vi "Build State Machine.vi"() -> ()   [LabVIEW 2019, in "VIPM.lvclass"]
uses:
  VIPM.lvclass
  <vilib>/Utility/sysdir.llb/System Directory Type.ctl
  <vilib>/Utility/file.llb/Read Delimited Spreadsheet (string).vi
  <vilib>/Utility/file.llb/Write Delimited Spreadsheet (string).vi
  <vilib>/JKI/VIPM API/VIPM API_vipm_api.lvlib
panel:
  out "Selected List":string
  in  "Publish":bool
  in  "Choose File":bool
  in  "Open Selected":bool
  in  "Preview All":bool
  in  "Build All":bool
  in  "Build Selected":bool
  in  "Preview Selected":bool
  out "Status":string
  in  "File List":i32(listbox)
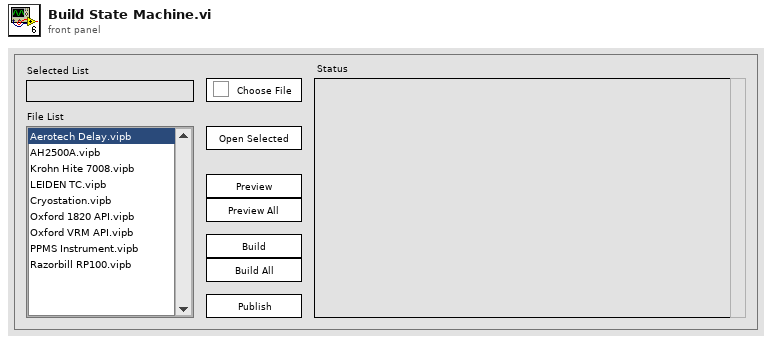
[diagram p1: front panel]
types:
  T1 = enum32{"Invalid", "Standard", "Closed", "Hidden", "Minimized", "Maximized"}
  T2 = enum32{"invalid app kind", "Development System", "Run Time System", "Student Edition", "Embedded LabVIEW", "Evaluation", "Custom"}
  T3 = enum8{"Enabled", "Disabled", "Disabled and Grayed Out"}
  T4 = cluster{"Core":cluster{"Current VI Reference":refnum<vi>, "Close Panel on Exit?":bool}, "lvproj paths":path[], "vipb paths":path[], "vip paths":path[], "selected path":path, "config path":path}
  T5 = typedef "System Directory Type.ctl" = i32
  T6 = cluster{"Current VI Reference":refnum<vi>, "Close Panel on Exit?":bool}
  T7 = typedef "VIPM API_vipm_api.lvlib/VI Package Build Spec Data Cluster_vipm_api.ctl" = cluster{"Package Version":T8, "Product Name":string, "Company Name":string, "Author Name (Person or Company)":string, "Product Homepage (URL)":string, "Legal Copyright":string, "License Agreement Name":string, "Product Description Summary":string, "Product Description":string, "Release Notes - Change Log":string}
  T8 = typedef "VIPM API_vipm_api.lvlib/Version Info Cluster_vipm_api.ctl" = cluster{"major":u32, "minor":u32, "patch":u32, "build":u32}
  T9 = typedef "VIPM API_vipm_api.lvlib/Repository Info Cluster_vipm_api.ctl" = cluster{"Repository Name":string, "Repository Folder Location":path}
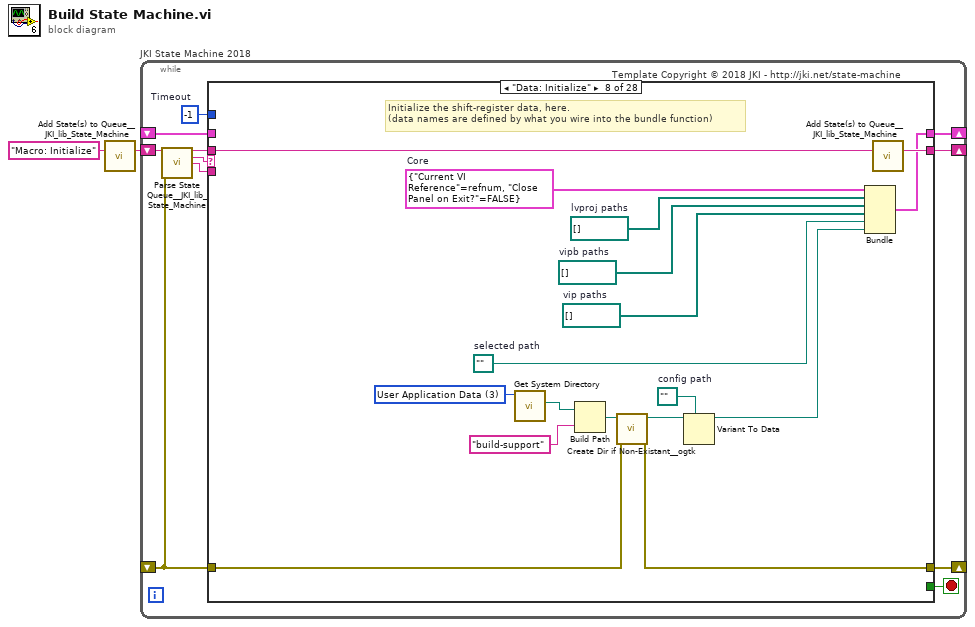
[diagram p0: block diagram]
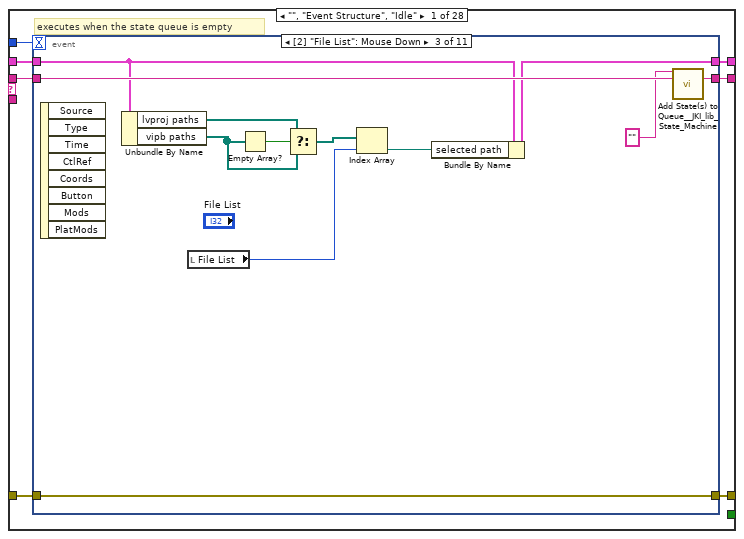
[diagram p2: hidden frame]
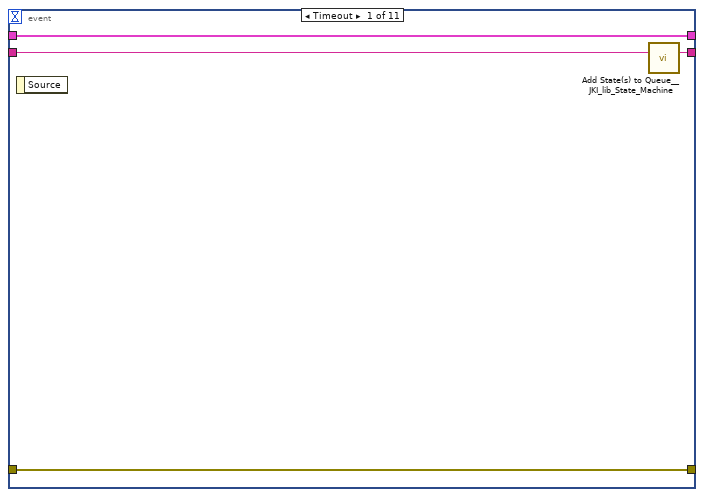
[diagram p3: hidden frame]
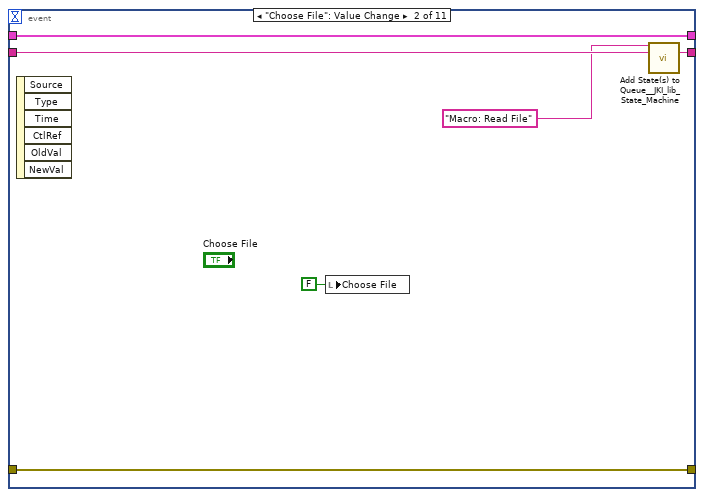
[diagram p4: hidden frame]
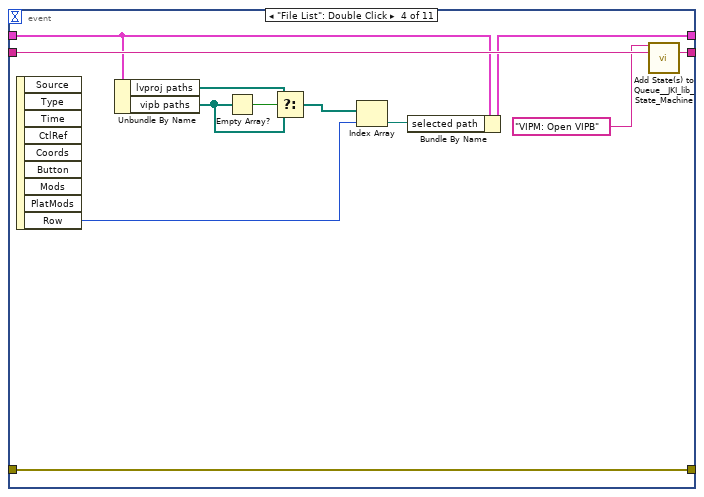
[diagram p5: hidden frame]
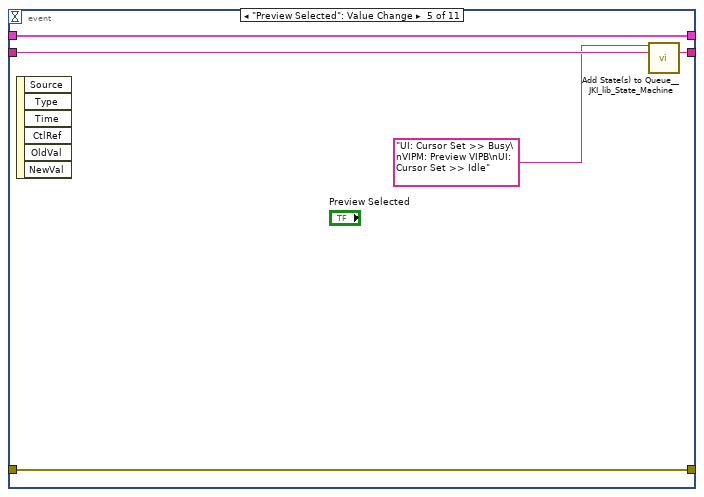
[diagram p6: hidden frame]
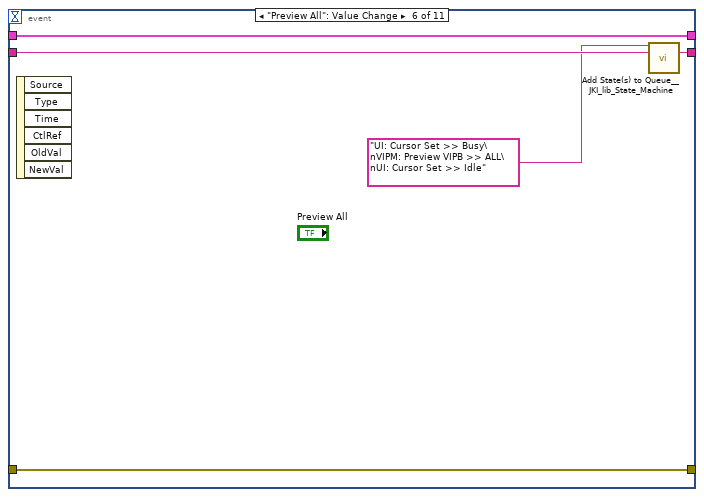
[diagram p7: hidden frame]
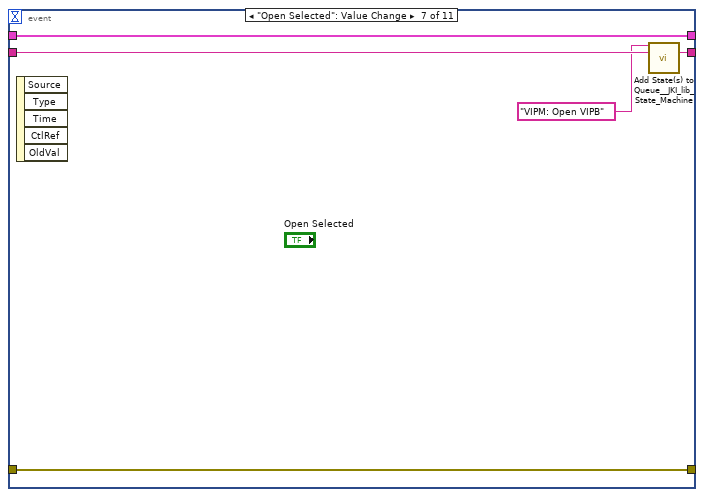
[diagram p8: hidden frame]
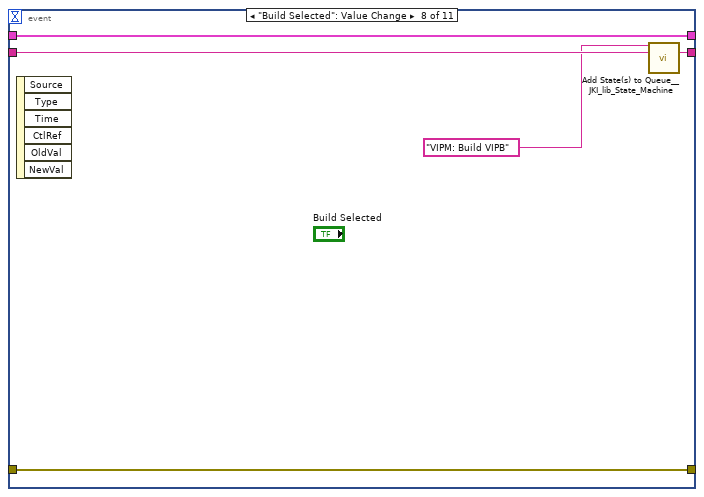
[diagram p9: hidden frame]
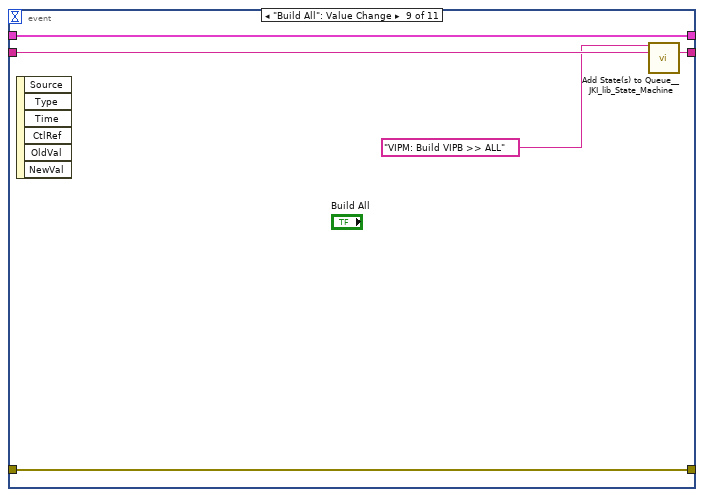
[diagram p10: hidden frame]
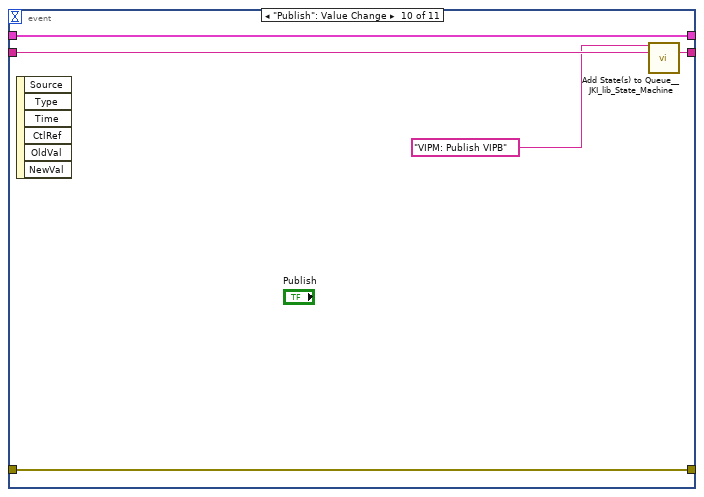
[diagram p11: hidden frame]
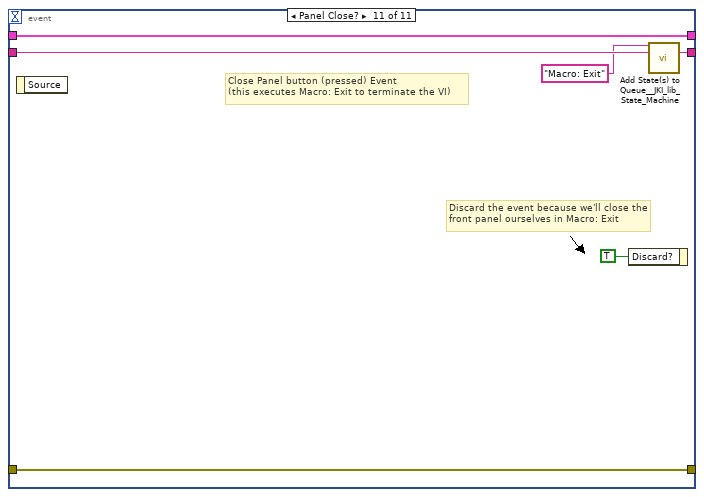
[diagram p12: hidden frame]
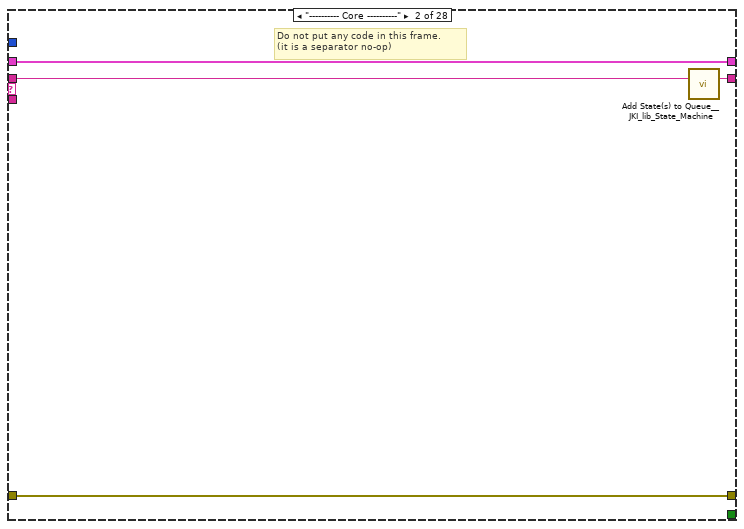
[diagram p13: hidden frame]
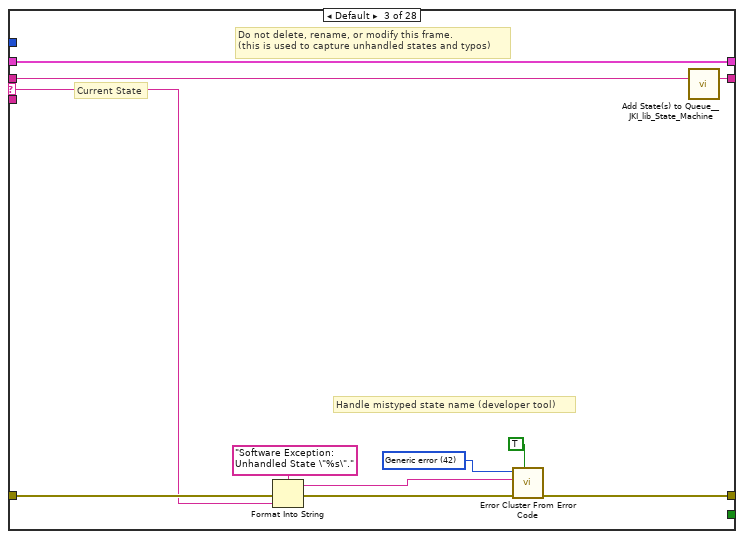
[diagram p14: hidden frame]
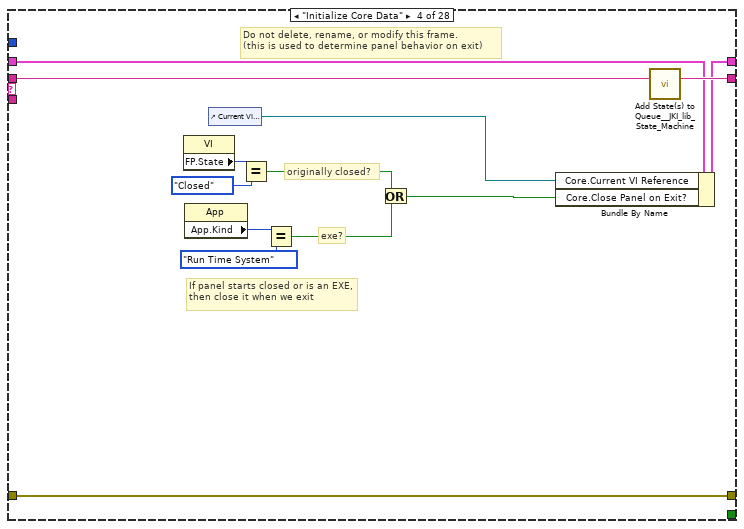
[diagram p15: hidden frame]
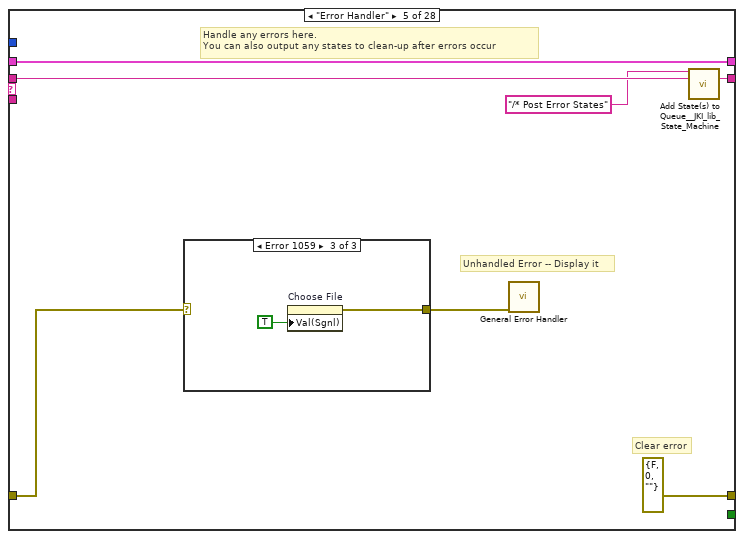
[diagram p16: hidden frame]
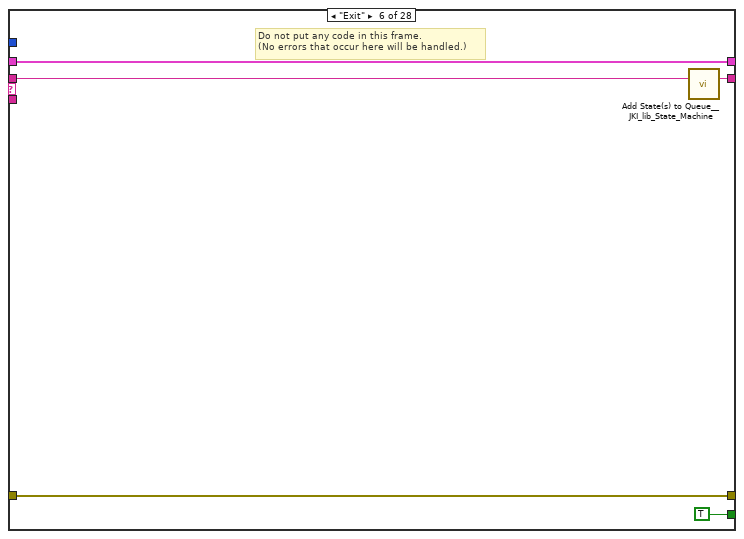
[diagram p19: hidden frame]
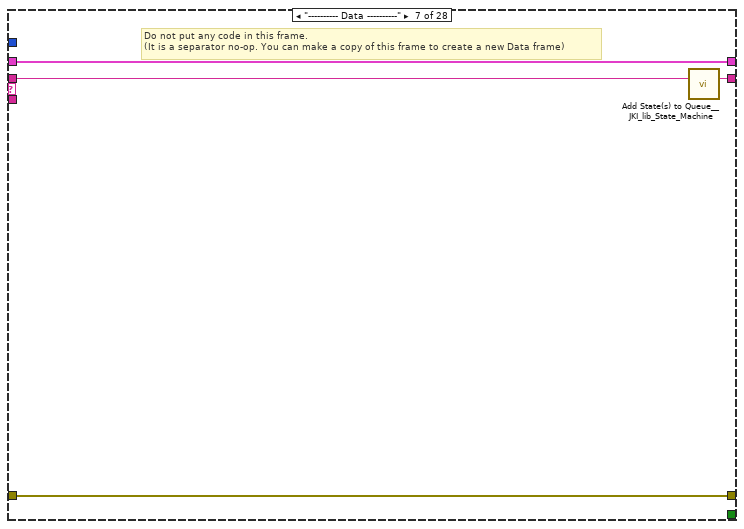
[diagram p20: hidden frame]
diagram:
  n1 = call <vilib>:"Add State(s) to Queue__JKI_lib_State_Machine.vi"("State(s) in (\"\")"="Macro: Initialize") -> ("States Out"=w2:string)  [unwired: 14 in]
  n2 = while "JKI State Machine 2018" {
    shift-right: [w6] -> _
    shift-left: _ -> [w5]
    shift-right: [w9] -> _
    shift-left: _ -> [w3]
    shift-right: [w8] -> _
    shift-left: w2 -> [w10]
    stop <- w7 stop-if-true
    w4 = -1  # Timeout
    # "Template Copyright © 2018 JKI - http://jki.net/state-machine"
    n3 = call <vilib>:"Parse State Queue__JKI_lib_State_Machine.vi"("State Queue"=w10, "Error In (no error)"=w3) -> ("Remaining States"=w12:string, "Current State"=w13:string, "Arguments"=w11:string)  [unwired: 11 in]
    n4 = case shown="\"Data: Initialize\"" w13 {
      selector: w13 -> [_ _ w95 _ _ _ _ _ _ _ _ _ _ _ _ _ _ _ _ _ _ _ _ _ _ _ _ _]
      tunnel: w12 -> [w20 w94 w99 w118 w125 w134 w138 w155 w161 w173 w186 w207 w226 w230 w236 w247 w264 w272 w283 w352 w357 w362 w372 w376 w389 w403 w426 w443]
      tunnel: w11 -> [_ _ _ _ _ _ _ _ _ _ _ _ _ _ _ _ _ w267 w277 _ _ _ _ _ _ w397 w412 _]
      tunnel: w5 -> [w18 w91 w97 w111 w122 w132 w135 _ w156 w165 w179 w204 w224 w227 w234 w244 w255 w270 w279 w349 w354 w359 w369 w373 w387 w400 w415 w437]
      tunnel: [w17 w92 w101 w115 errorcluster {"status"=FALSE, "code"=0, "source"=""} ("error out") w131 w136 w147 w157 w171 w176 w193 w220 w228 w233 w245 w262 w268 w280 w350 w355 w360 w370 w374 w382 w399 w418 w435] -> w9
      tunnel: w3 -> [w16 w92 w100 w115 w120 w131 w136 w146 w158 w171 w181 w202 w221 w228 w232 w245 w262 w269 w281 w350 w355 w360 w370 w374 w381 w398 w417 w434]
      tunnel: [w19 w93 w98 w117 w124 w133 w137 w154 w160 w172 w185 w206 w225 w229 w235 w246 w263 w271 w282 w351 w356 w361 w371 w375 w388 w402 w425 w442] -> w8
      tunnel: [_ _ _ _ _ TRUE _ _ _ _ _ _ _ _ _ _ _ _ _ _ _ _ _ _ _ _ _ _] -> w7
      tunnel: [w15 w91 w97 w116 w122 w132 w135 w153 w156 w166 w180 w205 w224 w227 w234 w244 w255 w270 w279 w349 w354 w359 w369 w373 w387 w400 w416 w437] -> w6
      tunnel: w4 -> [w14 _ _ _ _ _ _ _ _ _ _ _ _ _ _ _ _ _ _ _ _ _ _ _ _ _ _ _]
      frame "", "Event Structure", "Idle" {
        # "executes when the state queue is empty"
        n5 = event shown="[2] \"File List\": Mouse Down" {
          selector: _ -> [_ _ _ _ _ _ _ _ _ _ _]
          dyn-events: _ -> [_ _ _ _ _ _ _ _ _ _ _]
          timeout: w14 -> [_ _ _ _ _ _ _ _ _ _ _]
          tunnel: w20 -> [w24 w30 w42 w54 w59 w64 w69 w74 w79 w84 w90]
          tunnel: [w23 w29 w41 w53 w58 w63 w68 w73 w78 w83 w89] -> w19
          tunnel: w18 -> [w21 w25 w39 w44 w56 w61 w65 w71 w76 w81 w87]
          tunnel: [w22 w26 w40 w52 w57 w62 w67 w72 w77 w82 w88] -> w17
          tunnel: w16 -> [w22 w26 w40 w52 w57 w62 w67 w72 w77 w82 w88]
          tunnel: [w21 w25 w38 w51 w56 w61 w65 w71 w76 w81 w87] -> w15
          event Timeout {
            n6 = event-data() -> ()  [unwired: 1 in, 1 out]
            n7 = call <vilib>:"Add State(s) to Queue__JKI_lib_State_Machine.vi"("State(s) in (\"\")"=w24) -> ("States Out"=w23:string)  [unwired: 14 in]
          }
          event "Choose File": Value Change {
            n8 = event-data() -> ()  [unwired: 1 in, 6 out]
            n9 = local write "Choose File"(FALSE ("Choose File")) -> ()
            n10 = call <vilib>:"Add State(s) to Queue__JKI_lib_State_Machine.vi"("State(s) in Front (\"\")"="Macro: Read File" ("State(s) in Front (\"\")"), "State(s) in (\"\")"=w30) -> ("States Out"=w29:string)  [unwired: 13 in]
          }
          event "File List": Mouse Down {
            n11 = event-data() -> ()  [unwired: 1 in, 8 out]
            n12 = Unbundle By Name(w39) -> ("lvproj paths"=w33:path[], "vipb paths"=w31:path[])
            n13 = local read "File List"() -> (w35:i32)
            n14 = Empty Array?(array=w31) -> (empty?=w34:bool)
            n15 = Select(t=w33, s=w34, f=w31) -> (s? t:f=w32:path[])
            n16 = Index Array(array=w32, index=w35) -> (element=w37:path)
            n17 = Bundle By Name(cluster=w39, "selected path"=w37) -> (w38:T4)
            n18 = call <vilib>:"Add State(s) to Queue__JKI_lib_State_Machine.vi"("State(s) in Front (\"\")"="" ("State(s) in Front (\"\")"), "State(s) in (\"\")"=w42) -> ("States Out"=w41:string)  [unwired: 13 in]
          }
          event "File List": Double Click {
            n19 = event-data() -> ("Row"=w43:i32)  [unwired: 1 in, 8 out]
            n20 = Unbundle By Name(w44) -> ("lvproj paths"=w47:path[], "vipb paths"=w46:path[])
            n21 = Empty Array?(array=w46) -> (empty?=w48:bool)
            n22 = Select(t=w47, s=w48, f=w46) -> (s? t:f=w45:path[])
            n23 = Index Array(array=w45, index=w43) -> (element=w50:path)
            n24 = Bundle By Name(cluster=w44, "selected path"=w50) -> (w51:T4)
            n25 = call <vilib>:"Add State(s) to Queue__JKI_lib_State_Machine.vi"("State(s) in Front (\"\")"="VIPM: Open VIPB" ("State(s) in Front (\"\")"), "State(s) in (\"\")"=w54) -> ("States Out"=w53:string)  [unwired: 13 in]
          }
          event "Preview Selected": Value Change {
            n26 = event-data() -> ()  [unwired: 1 in, 6 out]
            n27 = call <vilib>:"Add State(s) to Queue__JKI_lib_State_Machine.vi"("State(s) in Front (\"\")"="UI: Cursor Set >> Busy\nVIPM: Preview VIPB\nUI: Cursor Set >> Idle" ("State(s) in Front (\"\")"), "State(s) in (\"\")"=w59) -> ("States Out"=w58:string)  [unwired: 13 in]
          }
          event "Preview All": Value Change {
            n28 = event-data() -> ()  [unwired: 1 in, 6 out]
            n29 = call <vilib>:"Add State(s) to Queue__JKI_lib_State_Machine.vi"("State(s) in Front (\"\")"="UI: Cursor Set >> Busy\nVIPM: Preview VIPB >> ALL\nUI: Cursor Set >> Idle" ("State(s) in Front (\"\")"), "State(s) in (\"\")"=w64) -> ("States Out"=w63:string)  [unwired: 13 in]
          }
          event "Open Selected": Value Change {
            n30 = event-data() -> ()  [unwired: 1 in, 5 out]
            n31 = call <vilib>:"Add State(s) to Queue__JKI_lib_State_Machine.vi"("State(s) in Front (\"\")"="VIPM: Open VIPB" ("State(s) in Front (\"\")"), "State(s) in (\"\")"=w69) -> ("States Out"=w68:string)  [unwired: 13 in]
          }
          event "Build Selected": Value Change {
            n32 = event-data() -> ()  [unwired: 1 in, 6 out]
            n33 = call <vilib>:"Add State(s) to Queue__JKI_lib_State_Machine.vi"("State(s) in Front (\"\")"="VIPM: Build VIPB" ("State(s) in Front (\"\")"), "State(s) in (\"\")"=w74) -> ("States Out"=w73:string)  [unwired: 13 in]
          }
          event "Build All": Value Change {
            n34 = event-data() -> ()  [unwired: 1 in, 6 out]
            n35 = call <vilib>:"Add State(s) to Queue__JKI_lib_State_Machine.vi"("State(s) in Front (\"\")"="VIPM: Build VIPB >> ALL" ("State(s) in Front (\"\")"), "State(s) in (\"\")"=w79) -> ("States Out"=w78:string)  [unwired: 13 in]
          }
          event "Publish": Value Change {
            n36 = event-data() -> ()  [unwired: 1 in, 6 out]
            n37 = call <vilib>:"Add State(s) to Queue__JKI_lib_State_Machine.vi"("State(s) in Front (\"\")"="VIPM: Publish VIPB" ("State(s) in Front (\"\")"), "State(s) in (\"\")"=w84) -> ("States Out"=w83:string)  [unwired: 13 in]
          }
          event Panel Close? {
            # "Discard the event because we'll close the front panel ourselves in Macro: Exit"
            # "Close Panel button (pressed) Event\n(this executes Macro: Exit to terminate the VI)"
            n38 = event-data() -> ()  [unwired: 1 in, 1 out]
            n39 = event-data("Discard?"=TRUE) -> ()  [unwired: 1 in, 1 out]
            n40 = call <vilib>:"Add State(s) to Queue__JKI_lib_State_Machine.vi"("State(s) in Front (\"\")"="Macro: Exit", "State(s) in (\"\")"=w90) -> ("States Out"=w89:string)  [unwired: 13 in]
          }
        }
      }
      frame "---------- Core ----------" {
        # "Do not put any code in this frame.\n(it is a separator no-op)"
        n41 = call <vilib>:"Add State(s) to Queue__JKI_lib_State_Machine.vi"("State(s) in (\"\")"=w94) -> ("States Out"=w93:string)  [unwired: 14 in]
      }
      frame Default {
        w104 = 42 items=["No error", "Argument error", "Memory is full", "Out of zone", "End of file", "File already open", "Generic file I/O error", "File not found", "File permission error", "Disk is full", "Duplicate path", "Too many files open", "System feature not enabled", "Resource file not found", "Cannot add resource", "Resource not found", "Image not found", "Image memory error", "Pen does not exist", "Config type invalid", "Config token not found", "Config parse error", "Config memory error", "Bad external code format", "Bad external code offset", "External code not present", "Null window", "Destroy window error", "Null menu", "Print aborted", "Bad print record", "Print driver error", "Windows error during printing", "Memory error during printing", "Print dialog error", "Generic print error", "Invalid device refnum", "Device not found", "Device parameter error", "Device unit error", "Cannot open device", "Device call aborted", "Generic error", "Cancelled by user", "Object ID too low", "Object ID too high", "Object not in heap", "Unknown heap", "Unknown object (invalid DefProc)", "Unknown object (DefProc not in table)", "Message out of range", "Invalid (null) method", "Unknown message", "Manager call not supported", "Bad address", "Network operation in progress", "Network operation timed out", "Connection is busy", "Network attribute not supported", "Network error", "Address in use", "System out of memory", "Connection aborted", "Connection refused", "Not connected", "Already connected", "Connection closed", "Initialization error (interapplication manager)", "Bad occurrence", "Wait on unbound occurrence handler", "Occurrence queue overflow", "Datalog type conflict", "Unused", "Unrecognized type (interapplication manager)", "Memory corrupt", "Failed to make temporary DLL", "Old CIN version", "Drag socket not found", "Failed to load drop-object", "Failed to register OLE object", "Failed to release OLE object", "Format specifier type mismatch", "Unknown format specifier", "Too few format specifiers", "Too many format specifiers", "Scan failed", "Newer CIN version", "Error converting to variant", "Runtime menu error", "Password tampered", "Variant attribute not found", "Incompatible variant data type", "Event data is not available", "Event Store is not present", "Occurrence is not found", "Event Queue is not created", "Event info is not available", "Refnum passed is NULL", "Error retrieving Class GUID", "Error retrieving CoClass GUID", "Error retrieving TypeLib GUID.", "Bad built application magic bytes.", "Specific driver is different from the specific driver associated with the Logical Name.", "There is no session opened to the class driver.", "Max Error", "MAX - Error with config objects", "MAX - Error loading configuration", "MAX - Group not supported"]
        # "Current State"
        # "Do not delete, rename, or modify this frame.\n(this is used to capture unhandled states and typos)"
        # "Handle mistyped state name (developer tool)"
        n42 = Format Into String(format string="Software Exception: Unhandled State \"%s\"." ("message"), error in=w100, w95) -> (resulting string=w103:string, error out=w102:errorcluster)  [unwired: 1 in]
        n43 = call <vilib>:"Error Cluster From Error Code.vi"("show call chain? (False)"=TRUE, "error in (no error)"=w102, "error message (\"\")"=w103, "error code (0)"=w104) -> ("error out"=w101:errorcluster)  [unwired: 5 in]
        n44 = call <vilib>:"Add State(s) to Queue__JKI_lib_State_Machine.vi"("State(s) in (\"\")"=w99) -> ("States Out"=w98:string)  [unwired: 14 in]
      }
      frame "Initialize Core Data" {
        # "Do not delete, rename, or modify this frame.\n(this is used to determine panel behavior on exit)"
        # "originally closed?"
        # "exe?"
        # "If panel starts closed or is an EXE, then close it when we exit"
        n45 = property class="VI"() -> ("FP.State"=w108:T1)  [unwired: 2 in, 2 out]
        n46 = property class="App"() -> ("App.Kind"=w114:T2)  [unwired: 2 in, 2 out]
        n47 = control-ref of="Current VI Reference"() -> (w109:refnum<vi>)
        n48 = Equal?(x=w108, y=T1."Closed" ("Front Panel Window:State")) -> (x = y?=w106:bool)
        n49 = Equal?(x=w114, y=T2."Run Time System" ("Application:Kind")) -> (x = y?=w112:bool)
        n50 = Or(x=w106, y=w112) -> (x .or. y?=w110:bool)
        n51 = Bundle By Name(cluster=w111, "Core.Current VI Reference"=w109, "Core.Close Panel on Exit?"=w110) -> (w116:T4)
        n52 = call <vilib>:"Add State(s) to Queue__JKI_lib_State_Machine.vi"("State(s) in (\"\")"=w118) -> ("States Out"=w117:string)  [unwired: 14 in]
      }
      frame "Error Handler" {
        # "Unhandled Error -- Display it"
        # "Handle any errors here.\nYou can also output any states to clean-up after errors occur"
        # "Clear error"
        n53 = case shown="Error 1059" w120 {
          selector: w120 -> [w126 w127 _]
          tunnel: [w126 w127 w128] -> w119
          frame No Error {
          }
          frame Default {
          }
          frame Error {
            n54 = property on="Choose File" class="Bool (strict)"("Val(Sgnl)"=TRUE) -> (error out=w128:errorcluster)  [unwired: 2 in, 1 out]
          }
        }
        n55 = call <vilib>:"General Error Handler.vi"("error in (no error)"=w119) -> ()  [unwired: 10 in, 5 out]
        n56 = call <vilib>:"Add State(s) to Queue__JKI_lib_State_Machine.vi"("State(s) in Front (\"\")"="/* Post Error States", "State(s) in (\"\")"=w125) -> ("States Out"=w124:string)  [unwired: 13 in]
      }
      frame "Exit" {
        # "Do not put any code in this frame.\n(No errors that occur here will be handled.)"
        n57 = call <vilib>:"Add State(s) to Queue__JKI_lib_State_Machine.vi"("State(s) in (\"\")"=w134) -> ("States Out"=w133:string)  [unwired: 14 in]
      }
      frame "---------- Data ----------" {
        # "Do not put any code in this frame.\n(It is a separator no-op. You can make a copy of this frame to create a new Data frame)"
        n58 = call <vilib>:"Add State(s) to Queue__JKI_lib_State_Machine.vi"("State(s) in (\"\")"=w138) -> ("States Out"=w137:string)  [unwired: 14 in]
      }
      frame "Data: Initialize" {
        w142 = T5 3 items=["User Home"=0, "User Desktop"=1, "User Documents"=2, "User Application Data"=3, "User Preferences"=4, "User Temporary"=5, "Public Documents"=6, "Public Application Data"=7, "Public Preferences"=8, "Public Cache"=13, "System Core Libraries"=9, "System Installed Libraries"=10, "Application Files"=11, "Boot Volume Root"=12] ("system directory type")
        w143 = path[] []  # lvproj paths
        w144 = path[] []  # vip paths
        w145 = path[] []  # vipb paths
        w149 = path ""  # config path
        w151 = path ""  # selected path
        w152 = T6 {"Current VI Reference"=refnum, "Close Panel on Exit?"=FALSE}  # Core
        # "Initialize the shift-register data, here.\n(data names are defined by what you wire into the bundle function)"
        n59 = call <vilib>:"Get System Directory.vi"("system directory type"=w142) -> ("system directory"=w140:path)  [unwired: 10 in]
        n60 = Build Path(base path=w140, name or relative path="build-support") -> (appended path=w139:path)
        n61 = call <userlib>:"Create Dir if Non-Existant__ogtk.vi"("error in (no error)"=w146, "Directory Path"=w139) -> ("error out"=w147:errorcluster, "dup Directory Path"=w148:path)  [unwired: 7 in, 1 out]
        n62 = Variant To Data(type=w149, Variant=w148) -> (data=w150:path)  [unwired: 1 in, 1 out]
        n63 = Bundle("Core"=w152, "lvproj paths"=w143, "vipb paths"=w145, "vip paths"=w144, "selected path"=w151, "config path"=w150) -> (w153:T4)  [unwired: 1 in]
        n64 = call <vilib>:"Add State(s) to Queue__JKI_lib_State_Machine.vi"("State(s) in (\"\")"=w155) -> ("States Out"=w154:string)  [unwired: 14 in]
      }
      frame "Data: Cleanup" {
        # "Cleanup any data and references, here.\n(this is called automatically, by the Macro: Exit)"
        n65 = Unbundle By Name(w156) -> ("Core.Current VI Reference"=w159:refnum<vi>)
        n66 = Close Reference(reference=w159, error in (no error)=w158) -> (error out=w157:errorcluster)
        n67 = call <vilib>:"Add State(s) to Queue__JKI_lib_State_Machine.vi"("State(s) in (\"\")"=w161) -> ("States Out"=w160:string)  [unwired: 14 in]
      }
      frame "Data: Update Listbox" {
        w162 = 0 ("Value (Signaling)")
        # "Do not put any code in this frame.\n(It is a separator no-op. You can make a copy of this frame to create a new Data frame)"
        n68 = Unbundle By Name(w165) -> ("lvproj paths"=w168:path[], "vipb paths"=w167:path[])
        n69 = Empty Array?(array=w167) -> (empty?=w169:bool)
        n70 = Select(t=w168, s=w169, f=w167) -> (s? t:f=w164:path[])
        n71 = for {
          tunnel: w164 -> [w175] mode=indexing
          tunnel: [w174] -> w170 mode=indexing
          n72 = Strip Path(path=w175) -> (name=w174:string)  [unwired: 1 out]
        }
        n73 = property on="File List" class="LstBox (strict)"("Item Names"=w170, "Val(Sgnl)"=w162) -> ()  [unwired: 2 in, 2 out]
        n74 = Index Array(array=w164, index=w162) -> (element=w163:path)
        n75 = Bundle By Name(cluster=w165, "selected path"=w163) -> (w166:T4)
        n76 = call <vilib>:"Add State(s) to Queue__JKI_lib_State_Machine.vi"("State(s) in (\"\")"=w173) -> ("States Out"=w172:string)  [unwired: 14 in]
      }
      frame "Data: Choose Config File" {
        # "Do not put any code in this frame.\n(It is a separator no-op. You can make a copy of this frame to create a new Data frame)"
        n77 = Unbundle By Name(w179) -> ("config path"=w184:path)
        n78 = call "File Dialog"("start path"=w184, "error in"=w181) -> ("selected path"=w183:path, "cancelled"=w178:bool, "error out"=w177:errorcluster)  [unwired: 10 in, 1 out]
        n79 = case shown="False" w178 {
          tunnel: w183 -> [w187 _]
          tunnel: [w191 _] -> w182
          tunnel: [w190 w192] -> w180
          tunnel: w179 -> [w189 w192]
          tunnel: w177 -> [w188 _]
          tunnel: [w188 _] -> w176
          frame False {
            n80 = Bundle By Name(cluster=w189, "config path"=w187) -> (w190:T4)
            n81 = Strip Path(path=w187) -> (name=w191:string)  [unwired: 1 out]
          }
          frame True {
          }
        }
        "Selected List" <- w182
        n82 = call <vilib>:"Add State(s) to Queue__JKI_lib_State_Machine.vi"("State(s) in (\"\")"=w186) -> ("States Out"=w185:string)  [unwired: 14 in]
      }
      frame "Data: Read Config File" {
        (unwired) 0 ("disabled index (col)")
        # "Do not put any code in this frame.\n(It is a separator no-op. You can make a copy of this frame to create a new Data frame)"
        n83 = Unbundle By Name(w204) -> ("config path"=w203:path)
        n84 = call-poly <vilib>:"Read Delimited Spreadsheet.vi"("file path (dialog if empty)"=w203, "error in (no error)"=w202, "transpose? (F)"=TRUE, "delimiter (\\t)"="\\n" ("delimiter (\\t)")) -> ("all rows"=w200:string[][], "error out"=w194:errorcluster)  [unwired: 6 in, 4 out]
        n85 = Index Array(array=w200) -> (element=w199:string[])  [unwired: 2 in]
        n86 = String To Path(string=w199) -> (path=w197:path[])
        n87 = for {
          tunnel: w197 -> [w216] mode=indexing
          tunnel: [w211] -> w196 mode=indexing if=w214
          tunnel: [w211] -> w195 mode=indexing if=w210
          tunnel: w194 -> [w209]
          tunnel: [w208] -> w193
          n88 = call <vilib>:"Get File Extension.vi"("error in (no error)"=w209, "file"=w216) -> ("error out"=w208:errorcluster, "lowercase file extension"=w212:string, "dup file"=w211:path)  [unwired: 5 in, 2 out]
          n89 = Equal?(x=w212, y="vipb") -> (x = y?=w214:bool)
          n90 = Equal?(x=w212, y="lvproj") -> (x = y?=w210:bool)
        }
        n91 = Bundle By Name(cluster=w204, "vipb paths"=w196, "lvproj paths"=w195) -> (w205:T4)
        n92 = call <vilib>:"Add State(s) to Queue__JKI_lib_State_Machine.vi"("State(s) in (\"\")"=w207) -> ("States Out"=w206:string)  [unwired: 14 in]
      }
      frame "Data: Write Config File" {
        # "Do not put any code in this frame.\n(It is a separator no-op. You can make a copy of this frame to create a new Data frame)"
        n93 = Unbundle By Name(w224) -> ("config path"=w219:path, "vipb paths"=w223:path[])
        n94 = Path To String(path=w223) -> (string=w222:string[])
        n95 = call-poly <vilib>:"Write Delimited Spreadsheet.vi"("file path (dialog if empty)"=w219, "1D data"=w222, "error in (no error)"=w221, "transpose? (no:F)"=TRUE, "delimiter (\\t)"="\\n" ("delimiter (\\t)")) -> ("error out"=w220:errorcluster)  [unwired: 9 in, 1 out]
        n96 = call <vilib>:"Add State(s) to Queue__JKI_lib_State_Machine.vi"("State(s) in (\"\")"=w226) -> ("States Out"=w225:string)  [unwired: 14 in]
      }
      frame "---------- UI ----------" {
        # "Do not put any code in this frame.\n(It is a separator no-op. You can make a copy of this frame to create a new UI frame)"
        n97 = call <vilib>:"Add State(s) to Queue__JKI_lib_State_Machine.vi"("State(s) in (\"\")"=w230) -> ("States Out"=w229:string)  [unwired: 14 in]
      }
      frame "UI: Initialize" {
        # "Initialize the User Interface, here.\n(this is called automatically, by the Macro: Init)"
        n98 = call <userlib>:"Fit VI window to Largest Dec__ogtk.vi"("error in (no error)"=w232) -> ("error out"=w233:errorcluster)  [unwired: 5 in, 1 out]
        n99 = local write "Status"("" ("Status")) -> ()
        n100 = call <vilib>:"Add State(s) to Queue__JKI_lib_State_Machine.vi"("State(s) in (\"\")"=w236) -> ("States Out"=w235:string)  [unwired: 14 in]
      }
      frame "UI: Disable Buttons" {
        # "Do not put any code in this frame.\n(It is a separator no-op. You can make a copy of this frame to create a new UI frame)"
        n101 = control-ref of="Open Selected"() -> (w237:refnum<vi>)
        n102 = control-ref of="Preview Selected"() -> (w243:refnum<vi>)
        n103 = control-ref of="Preview All"() -> (w242:refnum<vi>)
        n104 = control-ref of="Build Selected"() -> (w241:refnum<vi>)
        n105 = control-ref of="Build All"() -> (w240:refnum<vi>)
        n106 = control-ref of="Publish"() -> (w239:refnum<vi>)
        n107 = Build Array(w237, w243, w242, w241, w240, w239) -> (w238:refnum<vi>[])
        n108 = for {
          tunnel: w238 -> [w248] mode=indexing
          n109 = property class="Bool"(reference=w248, "DisabledEnum"=T3."Disabled and Grayed Out" ("Disabled")) -> ()  [unwired: 1 in, 2 out]
        }
        n110 = call <vilib>:"Add State(s) to Queue__JKI_lib_State_Machine.vi"("State(s) in (\"\")"=w247) -> ("States Out"=w246:string)  [unwired: 14 in]
      }
      frame "UI: Enable Buttons" {
        # "Do not put any code in this frame.\n(It is a separator no-op. You can make a copy of this frame to create a new UI frame)"
        n111 = Unbundle By Name(w255) -> ("vipb paths"=w256:path[])
        n112 = control-ref of="Open Selected"() -> (w254:refnum<vi>)
        n113 = control-ref of="Preview Selected"() -> (w261:refnum<vi>)
        n114 = control-ref of="Preview All"() -> (w260:refnum<vi>)
        n115 = control-ref of="Build Selected"() -> (w259:refnum<vi>)
        n116 = control-ref of="Build All"() -> (w258:refnum<vi>)
        n117 = control-ref of="Publish"() -> (w257:refnum<vi>)
        n118 = Empty Array?(array=w256) -> (empty?=w253:bool)
        n119 = Build Array(w254, w261, w260, w259, w258, w257) -> (w251:refnum<vi>[])
        n120 = Build Array(w254) -> (w252:refnum<vi>[])
        n121 = Select(t=w252, s=w253, f=w251) -> (s? t:f=w250:refnum<vi>[])
        n122 = for {
          tunnel: w250 -> [w265] mode=indexing
          n123 = property class="Bool"(reference=w265, "DisabledEnum"=T3."Enabled" ("Disabled")) -> ()  [unwired: 1 in, 2 out]
        }
        n124 = call <vilib>:"Add State(s) to Queue__JKI_lib_State_Machine.vi"("State(s) in (\"\")"=w264) -> ("States Out"=w263:string)  [unwired: 14 in]
      }
      frame "UI: Cursor Set" {
        # "Argument"
        # "Set and Unset Cursor Busy.\n(Usage: \"UI: Cursor Set >> Busy|Idle\")"
        n125 = case shown="\"Idle\", Default" w267 {
          tunnel: w269 -> [w274 w276]
          tunnel: [w273 w275] -> w268
          frame "Idle", Default {
            n126 = call <vilib>:"Unset Busy.vi"("error in (no error)"=w274) -> ("error out"=w273:errorcluster)  [unwired: 10 in]
          }
          frame "Busy" {
            n127 = call <vilib>:"Set Busy.vi"("error in (no error)"=w276) -> ("error out"=w275:errorcluster)  [unwired: 9 in, 1 out]
          }
        }
        n128 = call <vilib>:"Add State(s) to Queue__JKI_lib_State_Machine.vi"("State(s) in (\"\")"=w272) -> ("States Out"=w271:string)  [unwired: 14 in]
      }
      frame "UI: Front Panel State" {
        # "Argument"
        # "Set Front Panel Open or Closed\n(Usage: \"UI: Front Panel State >> Open|Close\")"
        n129 = Unbundle By Name(w279) -> ("Core.Current VI Reference"=w278:refnum<vi>)
        n130 = case shown="\"Minimize\", \"Minimized\"" w277 {
          tunnel: w281 -> [w289 w304 w315 w328 w341]
          tunnel: [w291 w305 w317 w330 w343] -> w280
          tunnel: w278 -> [w290 w302 w316 w329 w342]
          frame "Open", "Standard", Default {
            w284 = T1."Standard" ("State")
            n131 = property class="VI"(reference=w290, error in=w289) -> (reference out=w287:refnum<vi>, error out=w288:errorcluster, "FP.State"=w286:T1)
            n132 = Not Equal?(x=w286, y=w284) -> (x != y?=w285:bool)
            n133 = case shown="True" w285 {
              tunnel: [w295 w297] -> w291
              tunnel: w288 -> [w294 w297]
              tunnel: w287 -> [w293 _]
              tunnel: w284 -> [w292 _]
              frame True {
                n134 = invoke class="VI" method="FP.Open"(reference=w293, error in=w294, "Activate"=TRUE, "State"=w292) -> (error out=w295:errorcluster)  [unwired: 1 in, 4 out]
              }
              frame False {
              }
            }
          }
          frame "Close", "Closed" {
            n135 = property class="VI"(reference=w302, error in=w304) -> (reference out=w301:refnum<vi>, error out=w303:errorcluster, "FP.State"=w299:T1)
            n136 = Not Equal?(x=w299, y=T1."Closed" ("Front Panel Window:State")) -> (x != y?=w298:bool)
            n137 = case shown="True" w298 {
              tunnel: [w306 w309] -> w305
              tunnel: w303 -> [w306 w308]
              tunnel: w301 -> [_ w307]
              frame False {
              }
              frame True {
                n138 = invoke class="VI" method="FP.Close"(reference=w307, error in=w308) -> (error out=w309:errorcluster)  [unwired: 1 in, 2 out]
              }
            }
          }
          frame "Hidden", "Hide" {
            w310 = T1."Hidden" ("State")
            n139 = property class="VI"(reference=w316, error in=w315) -> (reference out=w313:refnum<vi>, error out=w314:errorcluster, "FP.State"=w312:T1)
            n140 = Not Equal?(x=w312, y=w310) -> (x != y?=w311:bool)
            n141 = case shown="True" w311 {
              tunnel: [w321 w322] -> w317
              tunnel: w314 -> [w320 w322]
              tunnel: w313 -> [w319 _]
              tunnel: w310 -> [w318 _]
              frame True {
                n142 = invoke class="VI" method="FP.Open"(reference=w319, error in=w320, "State"=w318) -> (error out=w321:errorcluster)  [unwired: 2 in, 4 out]
              }
              frame False {
              }
            }
          }
          frame "Minimize", "Minimized" {
            w323 = T1."Minimized" ("State")
            n143 = property class="VI"(reference=w329, error in=w328) -> (reference out=w326:refnum<vi>, error out=w327:errorcluster, "FP.State"=w325:T1)
            n144 = Not Equal?(x=w325, y=w323) -> (x != y?=w324:bool)
            n145 = case shown="True" w324 {
              tunnel: [w334 w335] -> w330
              tunnel: w327 -> [w333 w335]
              tunnel: w326 -> [w332 _]
              tunnel: w323 -> [w331 _]
              frame True {
                n146 = invoke class="VI" method="FP.Open"(reference=w332, error in=w333, "State"=w331) -> (error out=w334:errorcluster)  [unwired: 2 in, 4 out]
              }
              frame False {
              }
            }
          }
          frame "Maximize", "Maximized" {
            w336 = T1."Maximized" ("State")
            n147 = property class="VI"(reference=w342, error in=w341) -> (reference out=w339:refnum<vi>, error out=w340:errorcluster, "FP.State"=w338:T1)
            n148 = Not Equal?(x=w338, y=w336) -> (x != y?=w337:bool)
            n149 = case shown="True" w337 {
              tunnel: [w347 w348] -> w343
              tunnel: w340 -> [w346 w348]
              tunnel: w339 -> [w345 _]
              tunnel: w336 -> [w344 _]
              frame True {
                n150 = invoke class="VI" method="FP.Open"(reference=w345, error in=w346, "State"=w344) -> (error out=w347:errorcluster)  [unwired: 2 in, 4 out]
              }
              frame False {
              }
            }
          }
        }
        n151 = call <vilib>:"Add State(s) to Queue__JKI_lib_State_Machine.vi"("State(s) in (\"\")"=w283) -> ("States Out"=w282:string)  [unwired: 14 in]
      }
      frame "---------- Macro ----------" {
        # "Do not put any code in this frame.\n(It is a separator no-op. You can make a copy of this frame to create a new Macro frame)"
        n152 = call <vilib>:"Add State(s) to Queue__JKI_lib_State_Machine.vi"("State(s) in (\"\")"=w352) -> ("States Out"=w351:string)  [unwired: 14 in]
      }
      frame "Macro: Initialize" {
        w353 = "Data: Initialize\nInitialize Core Data\nUI: Initialize\nUI: Front Panel State >> Open\n\nMacro: Read File"  # Data: Initialize Initialize Core Data UI: Initialize UI: Front Panel State >> Open  Macro: Read File
        # "Initialization Macro\n(This is called once, when the VI starts)"
        n153 = call <vilib>:"Add State(s) to Queue__JKI_lib_State_Machine.vi"("State(s) in Front (\"\")"=w353, "State(s) in (\"\")"=w357) -> ("States Out"=w356:string)  [unwired: 13 in]
      }
      frame "Macro: Read File" {
        w358 = "UI: Cursor Set >> Busy\nUI: Disable Buttons\nData: Choose Config File\nData: Read Config File\nData: Update Listbox\nUI: Enable Buttons\nUI: Cursor Set >> Idle"  # UI: Cursor Set >> Busy UI: Disable Buttons Data: Choose Config File Data: Read Config File Data: Update Listbox UI: Enable Buttons UI: Cursor Set >> Idle
        # "Initialization Macro\n(This is called once, when the VI starts)"
        n154 = call <vilib>:"Add State(s) to Queue__JKI_lib_State_Machine.vi"("State(s) in Front (\"\")"=w358, "State(s) in (\"\")"=w362) -> ("States Out"=w361:string)  [unwired: 13 in]
      }
      frame "Macro: Exit" {
        # "Exit Macro\n(This is called once, when the VI exits)"
        n155 = Unbundle By Name(w369) -> ("Core.Close Panel on Exit?"=w368:bool)
        n156 = Select(t="UI: Front Panel State >> Close", s=w368, f="") -> (s? t:f=w365:string)
        n157 = call <vilib>:"Add State(s) to Queue__JKI_lib_State_Machine.vi"("State(s) in (\"\")"=w365, "State(s) at Back (\"\")"="Data: Cleanup\nExit") -> ("States Out"=w363:string)  [unwired: 13 in]
        n158 = call <vilib>:"Add State(s) to Queue__JKI_lib_State_Machine.vi"("State(s) in Front (\"\")"=w363, "State(s) in (\"\")"=w372) -> ("States Out"=w371:string)  [unwired: 13 in]
      }
      frame "---------- VIPM ----------" {
        # "Template Separator\n(You can make a copy of, or modify, this frame)"
        n159 = call <vilib>:"Add State(s) to Queue__JKI_lib_State_Machine.vi"("State(s) in (\"\")"=w376) -> ("States Out"=w375:string)  [unwired: 14 in]
      }
      frame "VIPM: Open VIPB" {
        # "Your code here.\n(You can make a copy of, or modify, this frame)"
        n160 = Unbundle By Name(w387) -> ("selected path"=w377:path)
        n161 = Format Into String(format string="cmd /c explorer.exe \"%s\"", error in=w381, w377) -> (resulting string=w385:string, error out=w383:errorcluster)  [unwired: 1 in]
        n162 = Strip Path(path=w377) -> (name=w379:string)  [unwired: 1 out]
        n163 = call <vilib>:"System Exec.vi"("run minimized? (F)"=TRUE, "error in (no error)"=w383, "command line"=w385) -> ("error out"=w382:errorcluster)  [unwired: 5 in, 3 out]
        n164 = Format Into String(format string="Opening \"%s\"...", w379) -> (resulting string=w380:string)  [unwired: 2 in, 1 out]
        n165 = local write "Status"(w380) -> ()
        n166 = call <vilib>:"Add State(s) to Queue__JKI_lib_State_Machine.vi"("State(s) in (\"\")"=w389) -> ("States Out"=w388:string)  [unwired: 14 in]
      }
      frame "VIPM: Preview VIPB" {
        # "Your code here.\n(You can make a copy of, or modify, this frame)"
        n167 = Equal?(x=w397, y="ALL") -> (x = y?=w390:bool)
        n168 = Unbundle By Name(w400) -> ("vipb paths"=w392:path[], "selected path"=w394:path)
        n169 = Build Array(w394) -> (w391:path[])
        n170 = Select(t=w392, s=w390, f=w391) -> (s? t:f=w393:path[])
        n171 = for {
          tunnel: w393 -> [w407] mode=indexing
          tunnel: [w410] -> w399
          tunnel: w398 -> [w409]
          tunnel: [w408] -> w395 mode=indexing
          n172 = Strip Path(path=w407) -> (name=w404:string)  [unwired: 1 out]
          n173 = Format Into String(format string="Reading \"%s\"...", w404) -> (resulting string=w406:string)  [unwired: 2 in, 1 out]
          n174 = call <vilib>:"Read VI Package Build Spec_vipm_api.vi"("error in (no error)"=w409, "Path to VIPB File"=w407) -> ("error out"=w410:errorcluster, "VI Package Build Spec Data"=w408:T7)  [unwired: 8 in]
          n175 = local write "Status"(w406) -> ()
        }
        n176 = call "Format Build Spec Summary.vi"("Build Spec [] in"=w395) -> ("VIPB Preview"=→"Status":string)  [unwired: 10 in]
        n177 = call <vilib>:"Add State(s) to Queue__JKI_lib_State_Machine.vi"("State(s) in (\"\")"=w403) -> ("States Out"=w402:string)  [unwired: 14 in]
      }
      frame "VIPM: Build VIPB" {
        # "Template Separator\n(You can make a copy of, or modify, this frame)"
        n178 = Equal?(x=w412, y="ALL") -> (x = y?=w419:bool)
        n179 = Unbundle By Name(w415) -> ("vipb paths"=w421:path[], "selected path"=w423:path)
        n180 = Build Array(w423) -> (w420:path[])
        n181 = Select(t=w421, s=w419, f=w420) -> (s? t:f=w422:path[])
        n182 = for {
          tunnel: w422 -> [w427] mode=indexing
          tunnel: [w433] -> w418
          tunnel: w417 -> [w432]
          tunnel: [w431] -> w414 mode=indexing
          n183 = Strip Path(path=w427) -> (name=w428:string)  [unwired: 1 out]
          n184 = Format Into String(format string="Building \"%s\"...", w428) -> (resulting string=w430:string)  [unwired: 2 in, 1 out]
          n185 = local write "Status"(w430) -> ()
          n186 = call <vilib>:"Build VI Package_vipm_api.vi"("error in (no error)"=w432, "Path to VIPB File"=w427) -> ("error out"=w433:errorcluster, "Build Output"=w431:path)  [unwired: 8 in]
        }
        n187 = call <vilib>:"Build State String with Arguments__JKI_lib_State_Machine.vi"("Arguments (\"\")"=w412, "State"="VIPM: Preview VIPB" ("State(s) in Front (\"\")")) -> ("State with Arguments"=w413:string)  [unwired: 4 in]
        n188 = Bundle By Name(cluster=w415, "vip paths"=w414) -> (w416:T4)
        n189 = call <vilib>:"Add State(s) to Queue__JKI_lib_State_Machine.vi"("State(s) in Front (\"\")"=w413, "State(s) in (\"\")"=w426) -> ("States Out"=w425:string)  [unwired: 13 in]
      }
      frame "VIPM: Publish VIPB" {
        # "Template Separator\n(You can make a copy of, or modify, this frame)"
        n190 = Unbundle By Name(w437) -> ("vip paths"=w436:path[])
        n191 = call <vilib>:"List VIPM Managed Repositories_vipm_api.vi"("error in (no error)"=w434) -> ("Managed Repositories Info"=w438:T9[], "error out"=w439:errorcluster)  [unwired: 13 in]
        n192 = Index Array(array=w438) -> (element=w440:T9)  [unwired: 1 in]
        n193 = Unbundle By Name(w440) -> ("Repository Name"=w441:string)
        n194 = call <vilib>:"Publish VI Packages to Repository_vipm_api.vi"("error in (no error)"=w439, "Repository Name"=w441, "Packages to publish to Repository Library (vip,ogp)"=w436) -> ("error out"=w435:errorcluster)  [unwired: 7 in, 1 out]
        n195 = call <vilib>:"Add State(s) to Queue__JKI_lib_State_Machine.vi"("State(s) in (\"\")"=w443) -> ("States Out"=w442:string)  [unwired: 14 in]
      }
    }
  }
